vi "SP Format Fundamental Value for Display (scalar).vi"(4 "Format":T1, 5 "Stored Value (0, linear)":dbl) -> (1 "Display Value":dbl)   [LabVIEW 2011]
uses:
  TypeDefs/SP Format.ctl
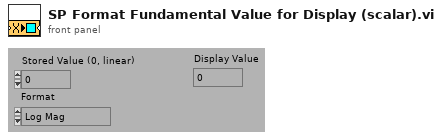
[diagram p1: front panel]
types:
  T1 = typedef "SP Format.ctl" = enum16{"Log Mag", "Lin Mag", "SWR", "Phase", "Expanded Phase", "Delay", "Insertion Loss", "Isolation", "Return Loss"}
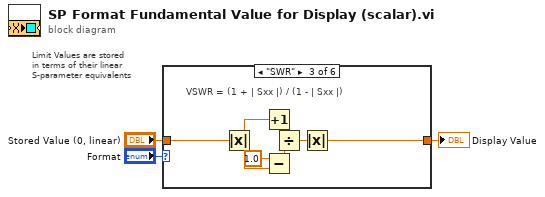
[diagram p0: block diagram]
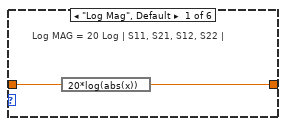
[diagram p2: hidden frame]
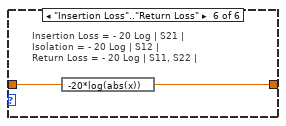
[diagram p6: hidden frame]
diagram:
  # "Limit Values are stored\nin terms of their linear\nS-parameter equivalents"
  n1 = case shown="\"SWR\"" "Format" {
    tunnel: [w4 w6 w7 w14 w15 w16] -> w1
    tunnel: "Stored Value (0, linear)" -> [w5 w6 w11 w14 w15 w17]
    frame "Log Mag", Default {
      # "Log MAG = 20 Log | S11, S21, S12, S22 |"
      n2 = expression code="20*log(abs(x))"(w5) -> (w4:dbl)
    }
    frame "Lin Mag" {
    }
    frame "SWR" {
      # "VSWR = (1 + | Sxx |) / (1 - | Sxx |)"
      n3 = Absolute Value(x=w11) -> (abs(x)=w8:dbl)
      n4 = Increment(x=w8) -> (x+1=w13:dbl)
      n5 = Subtract(x=1.0, y=w8) -> (x-y=w10:dbl)
      n6 = Divide(x=w13, y=w10) -> (x/y=w9:dbl)
      n7 = Absolute Value(x=w9) -> (abs(x)=w7:dbl)
    }
    frame "Phase", "Expanded Phase" {
    }
    frame "Delay" {
      # "Group Delay scalar quantities come straight from\nthe user and are saved in units of seconds..."
    }
    frame "Insertion Loss".."Return Loss" {
      # "Insertion Loss = - 20 Log | S21 |\nIsolation = - 20 Log | S12 |\nReturn Loss = - 20 Log | S11, S22 |"
      n8 = expression code="-20*log(abs(x))"(w17) -> (w16:dbl)
    }
  }
  "Display Value" <- w1
